vi "Change Wavelength.vi"(7 "error in":errorcluster, 10 "GOTO":dbl format="%.3f") -> (0 "error out":errorcluster={"status"=TRUE, "code"=65, "source"="McP Timeout"}, 1 "CurrentPosition":dbl(knob) caption="Current Wavelength" min=550.0 max=600.0 scale=824.0..826.0 scale format="%.1f", 3 "Final nm":dbl)   [LabVIEW 2024]
doc: "McPherson 789A-3 controller Vi to control McPherson 2075 spectrometer through serial port. If running directly, you need to initialize the serial port and the spectrometer. During this process, if the scan velocity returns to be 0, the program is suspended. You need to change the velocity manually to unblock."
uses:
  Globals and TypeDefs/Type Definitions.llb/3 way Status.ctl
  Globals and TypeDefs/Type Definitions.llb/McPherson Status.ctt
  Globals and TypeDefs/Error Categories.ctt
  <vilib>/Utility/error.llb/DialogType.ctl
  Globals and TypeDefs/gStatus.vi
  Globals and TypeDefs/gSpectrometer.vi
  Instance          10 25Saved   Change Wavelength .vi
panel:
  in  "Case Constant\n(See Context Help)":bool
  in  "Reset":bool
  in  "Time-out limit (s)":dbl=60.0
  out "ChangeWL Status":T1(ring)
  in  "stop":bool
  in  "Tolerance (WL)":dbl=0.01 min=0.0001 max=1.0 step=0.0001 format="%.3f"
  out "msec":u32
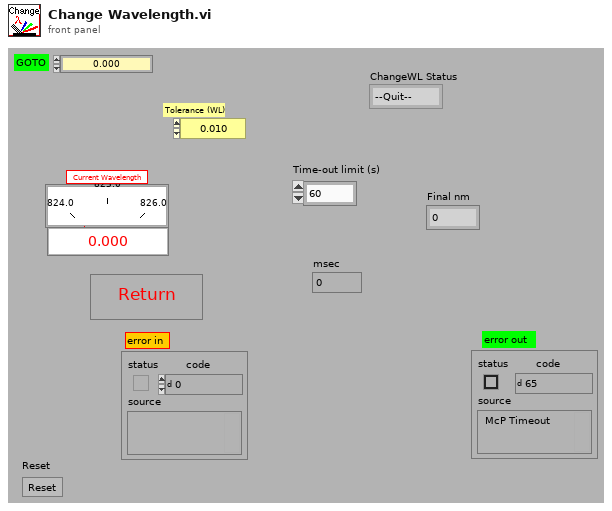
[diagram p1: front panel]
types:
  T1 = enum16{"--Quit--", "Read Initial Status", "Set New Field", "Check Field Value"}
  T2 = typedef "3 way Status.ctl" = u8
  T3 = enum16{"--Quit--", "Read Initial Status", "Set New Field", "Check Field Value", "Done"}
  T4 = typedef "McPherson Status.ctt" = enum8{"--Quit--", "Error", "Initialization", "Standby", "Start Slew", "-Slew", "+Slew", "Slew Done", "Start Scan", "-Slew to Start", "+Slew to Start", "Scanning", "Scan Done", "Scan Pause", "Slew Pause", "Cancel", "Update Z0", "Sleep"}
  T5 = enum8{"Initialization Error", "Command Error", "Parameter Error", "Overflow Error", "Time-out Error", "Misc Error", "User cancel"}
  T6 = typedef "Error Categories.ctt" = enum8{"General", "CCD-256x1024", "CCD-1340x400", "InGaAs PDA", "McPherson 2075", "Magnetic Field", "Temperature Control", "Other"}
  T7 = typedef "DialogType.ctl" = u16
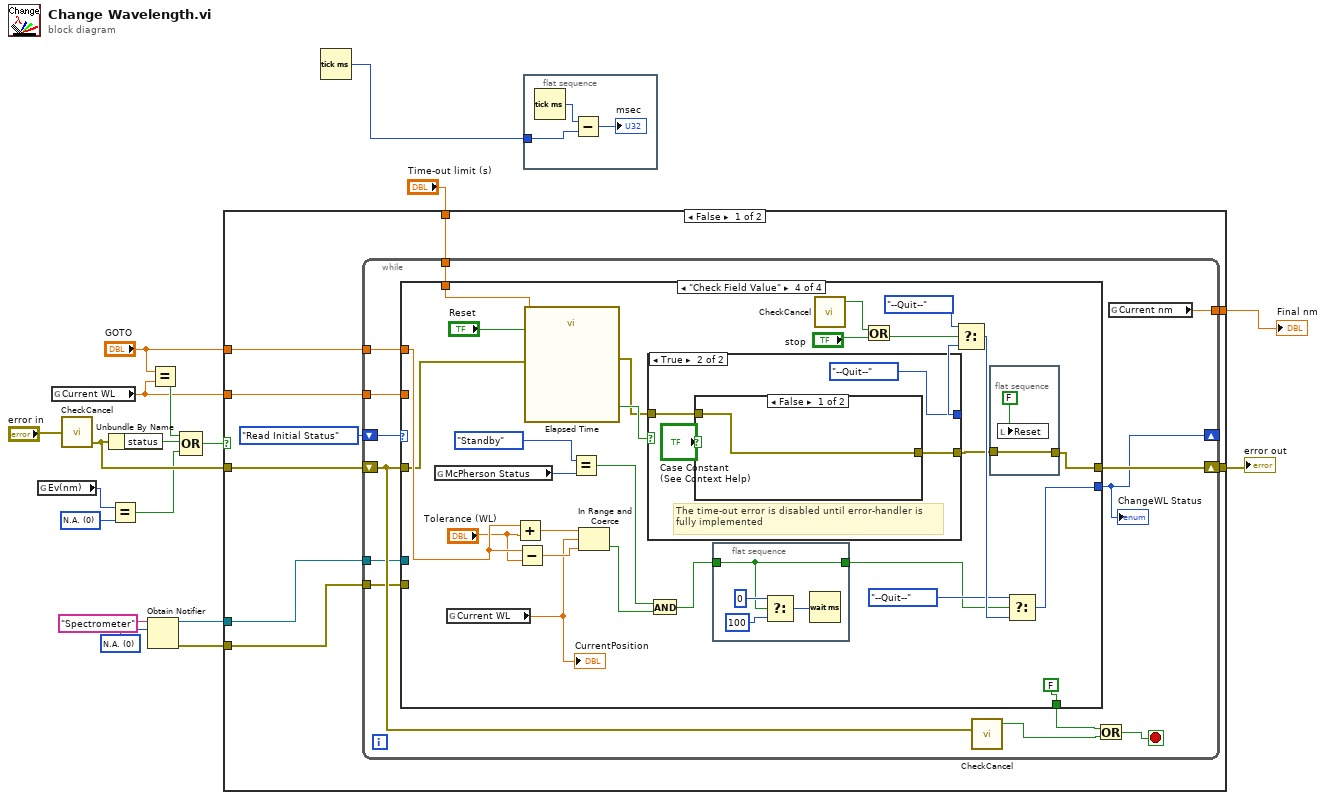
[diagram p0: block diagram]
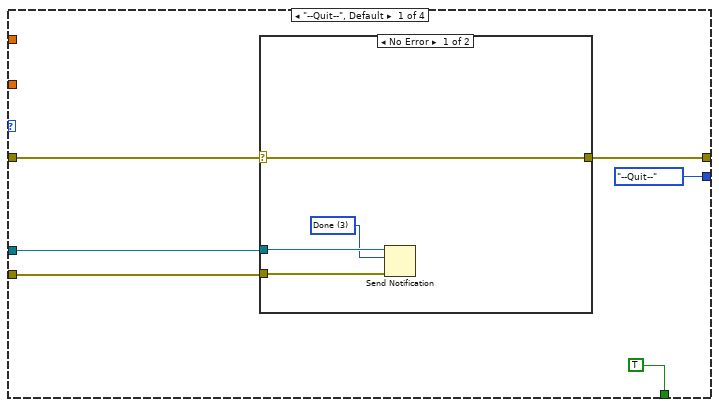
[diagram p2: hidden frame]
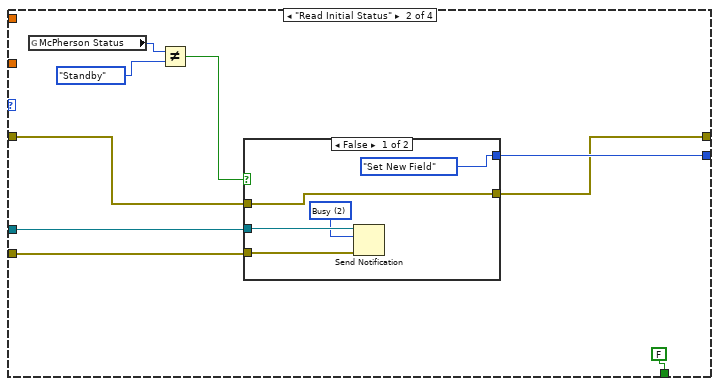
[diagram p4: hidden frame]
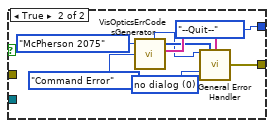
[diagram p5: hidden frame]
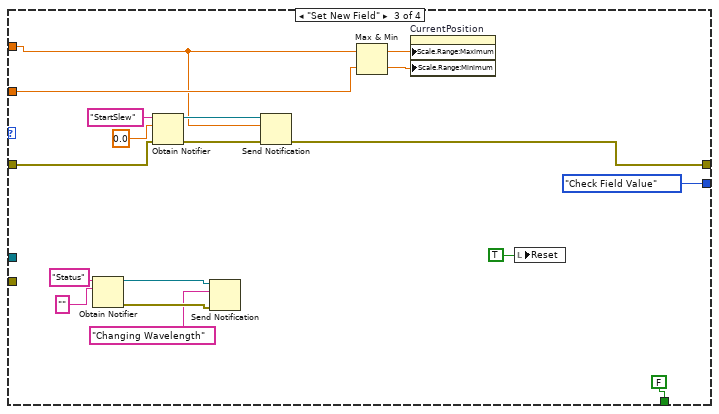
[diagram p6: hidden frame]
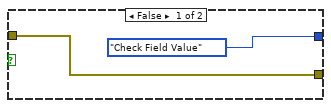
[diagram p7: hidden frame]
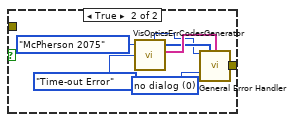
[diagram p8: hidden frame]
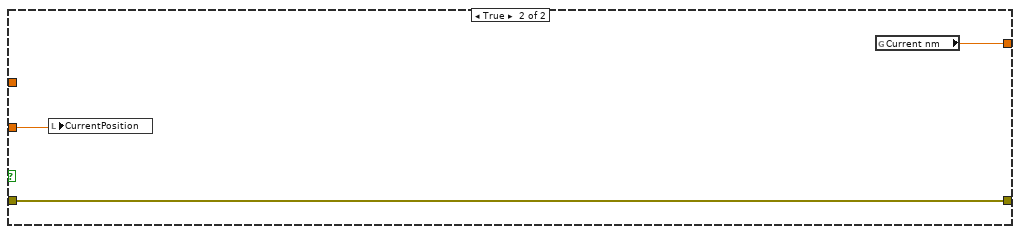
[diagram p9: hidden frame]
diagram:
  w13 = T2 0 items=["N.A.", "OK", "Busy", "Done"] ("Saving")
  w17 = T2 0 items=["N.A.", "OK", "Busy", "Done"] ("y")
  n1 = global read "gStatus.vi" "Ev(nm)"() -> (w16:T2)
  n2 = global read "gSpectrometer.vi" "Current WL"() -> (w4:dbl)
  n3 = call "CheckCancel.vi"("error in (no error)"="error in") -> ("error out"=w15:errorcluster)  [unwired: 1 in, 1 out]
  n4 = Unbundle By Name(w15) -> ("status"=w7:bool)
  n5 = Equal?(x=w16, y=w17) -> (x = y?=w6:bool)
  n6 = Obtain Notifier(name (unnamed)="Spectrometer", notification data type=w13) -> (notifier out=w12:refnum<notifier>, error out=w11:errorcluster)  [unwired: 2 in, 1 out]
  n7 = Equal?(x="GOTO", y=w4) -> (x = y?=w8:bool)
  n8 = Compound Arithmetic op=OR(w8, w7, w6) -> (w9:bool)
  n9 = case shown="False" w9 {
    tunnel: w15 -> [w27 w141]
    tunnel: [w26 w141] -> w3
    tunnel: w12 -> [w25 _]
    tunnel: w11 -> [w24 _]
    tunnel: "GOTO" -> [w23 _]
    tunnel: w4 -> [w22 w140]
    tunnel: "Time-out limit (s)" -> [w21 _]
    tunnel: [w19 w139] -> w1
    frame False {
      n10 = while {
        shift-right: [w29] -> _
        shift-left: T3."Read Initial Status" ("ChangeField Status") -> [w40]
        shift-right: [w39] -> w26
        shift-left: w27 -> [w34]
        tunnel: w23 -> [w38]
        tunnel: w25 -> [w33]
        tunnel: w24 -> [w32]
        tunnel: w22 -> [w31]
        tunnel: w21 -> [w30]
        tunnel: [w28] -> w19
        stop <- w37 stop-if-true
        n11 = case shown="\"Check Field Value\"" w40 {
          tunnel: w34 -> [w44 w56 w85 w96]
          tunnel: [w43 w55 w81 w97] -> w39
          tunnel: w38 -> [_ _ w82 w107]
          tunnel: [T3."--Quit--" ("ChangeField Status") w60 T3."Check Field Value" ("ChangeField Status") w113] -> w29
          tunnel: [TRUE FALSE FALSE FALSE] -> w36
          tunnel: w33 -> [w42 w58 _ _]
          tunnel: w32 -> [w41 w57 _ _]
          tunnel: w31 -> [_ _ w88 _]
          tunnel: w30 -> [_ _ _ w101]
          frame "--Quit--", Default {
            n12 = case shown="No Error" w44 {
              selector: w44 -> [w47 w51]
              tunnel: [w47 w51] -> w43
              tunnel: w42 -> [w50 _]
              tunnel: w41 -> [w49 _]
              frame No Error {
                w48 = T2 3 items=["N.A.", "OK", "Busy", "Done"] ("H(T)")
                n13 = Send Notification(notification=w48, notifier=w50, error in (no error)=w49) -> ()  [unwired: 2 out]
              }
              frame Error {
              }
            }
          }
          frame "Read Initial Status" {
            n14 = global read "gSpectrometer.vi" "McPherson Status"() -> (w54:T4)
            n15 = Not Equal?(x=w54, y=McPherson_Status.ctt."Standby") -> (x != y?=w52:bool)
            n16 = case shown="False" w52 {
              tunnel: [w65 w68] -> w55
              tunnel: w56 -> [w65 _]
              tunnel: [T3."Set New Field" ("ChangeField Status") T3."--Quit--" ("ChangeField Status")] -> w60
              tunnel: w58 -> [w63 _]
              tunnel: w57 -> [w62 _]
              frame False {
                w61 = T2 2 items=["N.A.", "OK", "Busy", "Done"] ("H(T)")
                n17 = Send Notification(notification=w61, notifier=w63, error in (no error)=w62) -> ()  [unwired: 2 out]
              }
              frame True {
                w73 = T7 0 items=["no dialog", "OK message", "continue or stop message", "OK message + warnings", "continue/stop + warnings"] ("type of dialog (OK msg:1)")
                n18 = call "VisOpticsErrCodesGenerator.vi"("NHMFL Visible Optics Error Type"=T5."Command Error", "NHMFL Visible Optics Error Categories"=Error_Categories.ctt."McPherson 2075") -> ("user-defined descriptions"=w72:string[], "User-defined Error Code"=w66:i32, "user-defined codes"=w71:i32[])  [unwired: 1 in, 3 out]
                n19 = call <vilib>:"General Error Handler.vi"("[error code] (0)"=w66, "[user-defined codes]"=w71, "[user-defined descriptions]"=w72, "type of dialog (OK msg:1)"=w73) -> ("error out"=w68:errorcluster)  [unwired: 7 in, 4 out]
              }
            }
          }
          frame "Set New Field" {
            n20 = Obtain Notifier(name (unnamed)="Status", notification data type="" ("Status")) -> (notifier out=w76:refnum<notifier>, error out=w75:errorcluster)  [unwired: 2 in, 1 out]
            n21 = Obtain Notifier(name (unnamed)="StartSlew", notification data type=0.0, error in (no error)=w85) -> (notifier out=w83:refnum<notifier>, error out=w84:errorcluster)  [unwired: 1 in, 1 out]
            n22 = Send Notification(notification="Changing Wavelength", notifier=w76, error in (no error)=w75) -> ()  [unwired: 2 out]
            n23 = Send Notification(notification=w82, notifier=w83, error in (no error)=w84) -> (error out=w81:errorcluster)  [unwired: 1 out]
            n24 = Max & Min(x=w82, y=w88) -> (max(x,y)=w90:dbl, min(x,y)=w89:dbl)
            n25 = property on="CurrentPosition" class="Knob (strict)"("Scale.Range:Maximum"=w90, "Scale.Range:Minimum"=w89) -> ()  [unwired: 2 in, 2 out]
            n26 = local write "Reset"(TRUE ("Reset")) -> ()
          }
          frame "Check Field Value" {
            n27 = global read "gSpectrometer.vi" "McPherson Status"() -> (w104:T4)
            n28 = global read "gSpectrometer.vi" "Current WL"() -> (w105:dbl)
            "CurrentPosition" <- w105
            n29 = Add(x=w107, y="Tolerance (WL)") -> (x+y=w109:dbl)
            n30 = Subtract(x=w107, y="Tolerance (WL)") -> (x-y=w108:dbl)
            n31 = call "Elapsed Time"("Time Target (s)"=w101, "Reset"="Reset", "error in (no error)"=w96) -> ("Time has Elapsed"=w100:bool, "error out"=w95:errorcluster)  [unwired: 9 in, 6 out]
            n32 = Equal?(x=McPherson_Status.ctt."Standby", y=w104) -> (x = y?=w102:bool)
            n33 = In Range and Coerce(upper limit=w109, x=w105, lower limit=w108) -> (In Range?=w116:bool)  [unwired: 1 out]
            n34 = case shown="True" w100 {
              tunnel: [w126 w130] -> w98
              tunnel: w95 -> [w126 w127]
              tunnel: [T3."Check Field Value" ("ChangeField Status") T3."--Quit--" ("ChangeField Status")] -> w118
              frame False {
              }
              frame True {
                # "The time-out error is disabled until error-handler is\nfully implemented"
                n35 = case shown="False" "Case Constant\n(See Context Help)" {
                  tunnel: [w131 w133] -> w130
                  tunnel: w127 -> [w131 _]
                  frame False {
                  }
                  frame True {
                    w138 = T7 0 items=["no dialog", "OK message", "continue or stop message", "OK message + warnings", "continue/stop + warnings"] ("type of dialog (OK msg:1)")
                    n36 = call "VisOpticsErrCodesGenerator.vi"("NHMFL Visible Optics Error Type"=T5."Time-out Error", "NHMFL Visible Optics Error Categories"=Error_Categories.ctt."McPherson 2075") -> ("user-defined descriptions"=w137:string[], "User-defined Error Code"=w132:i32, "user-defined codes"=w136:i32[])  [unwired: 1 in, 3 out]
                    n37 = call <vilib>:"General Error Handler.vi"("[error code] (0)"=w132, "[user-defined codes]"=w136, "[user-defined descriptions]"=w137, "type of dialog (OK msg:1)"=w138) -> ("error out"=w133:errorcluster)  [unwired: 7 in, 4 out]
                  }
                }
              }
            }
            n38 = And(x=w102, y=w116) -> (x .and. y?=w111:bool)
            n39 = flat-sequence {
              tunnel: [w121] -> w110
              tunnel: w111 -> [w121]
              frame #0 {
                n40 = Select(t=u32 0 ("milliseconds to wait"), s=w121, f=u32 100) -> (s? t:f=w123:u32)
                n41 = Wait (ms)(milliseconds to wait=w123) -> ()  [unwired: 1 out]
              }
            }
            n42 = call "CheckCancel.vi"() -> ("Cancelled"=w93:bool)  [unwired: 2 in, 1 out]
            n43 = Or(x=w93, y="stop") -> (x .or. y?=w94:bool)
            n44 = Select(t=T3."--Quit--" ("ChangeField Status"), s=w94, f=w118) -> (s? t:f=w115:T3)
            n45 = flat-sequence {
              tunnel: [w120] -> w97
              tunnel: w98 -> [w120]
              frame #0 {
                n46 = local write "Reset"(FALSE ("Reset")) -> ()
              }
            }
            n47 = Select(t=T3."--Quit--" ("f"), s=w110, f=w115) -> (s? t:f=w113:T3)
          }
        }
        "ChangeWL Status" <- w29
        n48 = call "CheckCancel.vi"("error in (no error)"=w34) -> ("Cancelled"=w35:bool)  [unwired: 1 in, 1 out]
        n49 = Or(x=w36, y=w35) -> (x .or. y?=w37:bool)
        n50 = global read "gSpectrometer.vi" "Current nm"() -> (w28:dbl)
      }
    }
    frame True {
      n51 = local write "CurrentPosition"(w140) -> ()
      n52 = global read "gSpectrometer.vi" "Current nm"() -> (w139:dbl)
    }
  }
  "error out" <- w3
  "Final nm" <- w1
  n53 = Tick Count (ms)() -> (millisecond timer value=w18:u32)
  n54 = flat-sequence {
    tunnel: w18 -> [w143]
    frame #0 {
      n55 = Tick Count (ms)() -> (millisecond timer value=w144:u32)
      n56 = Subtract(x=w144, y=w143) -> (x-y=→"msec":u32)
    }
  }
